vi "WaveGeneratorSelect.vi"(0 "Serial port name":refnum<visa-resource-name>, 2 "start commands":string[](array[string]), 3 "stop commands":string[](array[string])) -> (6 "waveform buffer":T1, 8 "error out":errorcluster)   [LabVIEW 2014]
uses:
  <vilib>/Instr/_visa.llb/VISA Flush IO Buffer Mask.ctl
  <vilib>/Instr/_visa.llb/VISA Configure Serial Port (Instr).vi
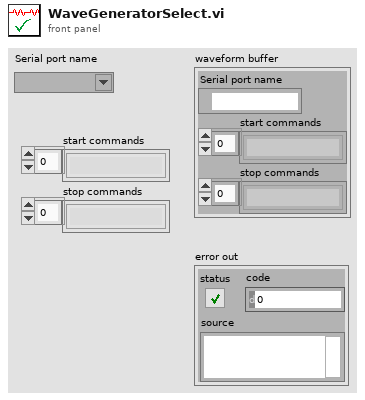
[diagram p1: front panel]
types:
  T1 = cluster{"Serial port name":refnum<visa-resource-name>, "start commands":string[], "stop commands":string[]}
  T2 = typedef "VISA Flush IO Buffer Mask.ctl" = u16
  T3 = cluster{"VISA resource name out":refnum<visa-resource-name>, "start commands":string[], "stop commands":string[]}
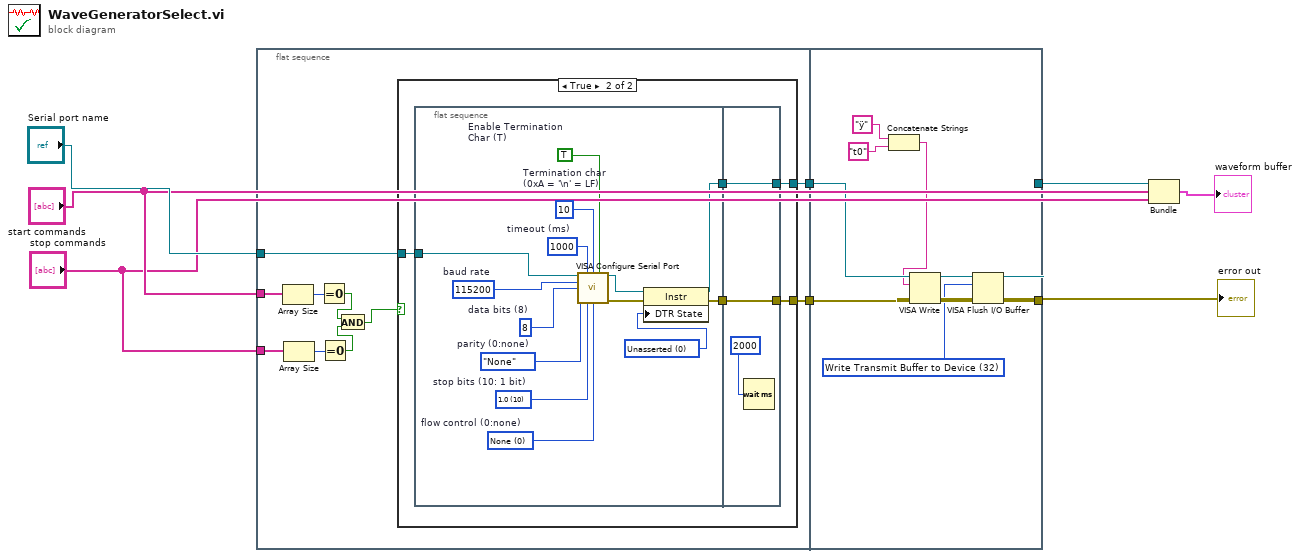
[diagram p0: block diagram]
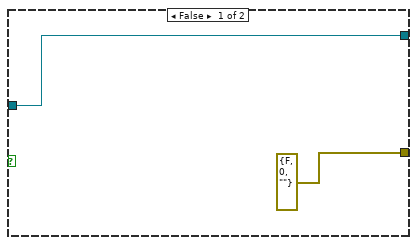
[diagram p2: hidden frame]
diagram:
  n1 = flat-sequence {
    tunnel: "Serial port name" -> [w10]
    tunnel: "start commands" -> [w14]
    tunnel: "stop commands" -> [w13]
    tunnel: [w12] -> w2
    tunnel: [w11] -> w1
    tunnel: [w44] -> w3
    tunnel: [w46] -> w4
    tunnel: w2 -> [w51]
    tunnel: w1 -> [w52]
    frame #0 {
      n2 = Array Size(array=w14) -> (size(s)=w18:i32)
      n3 = Array Size(array=w13) -> (size(s)=w17:i32)
      n4 = Equal To 0?(x=w18) -> (x = 0?=w15:bool)
      n5 = Equal To 0?(x=w17) -> (x = 0?=w16:bool)
      n6 = And(x=w15, y=w16) -> (x .and. y?=w9:bool)
      n7 = case shown="True" w9 {
        tunnel: [w20 w25] -> w12
        tunnel: [errorcluster {"status"=FALSE, "code"=0, "source"=""} ("error constant") w24] -> w11
        tunnel: w10 -> [w20 w23]
        frame False {
        }
        frame True {
          n8 = flat-sequence {
            tunnel: w23 -> [w26]
            tunnel: [w29] -> w22
            tunnel: [w28] -> w21
            tunnel: [w41] -> w24
            tunnel: [w42] -> w25
            tunnel: w22 -> [w42]
            tunnel: w21 -> [w41]
            frame #0 {
              w27 = i16 0 items=["Unknown"=-1, "Unasserted"=0, "Asserted"=1] ("Serial Settings:Modem Line Settings:Line DTR State")
              w32 = TRUE  # Enable Termination Char (T)
              w33 = u8 10  # Termination char (0xA = '\n' = LF)
              w34 = u16 0 items=["None", "XON/XOFF", "RTS/CTS", "XON/XOFF & RTS/CTS", "DTR/DSR", "XON/XOFF & DTR/DSR"]  # flow control (0:none)
              w35 = u16 10 items=["1.0"=10, "1.5"=15, "2.0"=20]  # stop bits (10: 1 bit)
              w36 = u32 1000  # timeout (ms)
              w37 = enum16{"None", "Odd", "Even", "Mark", "Space"}."None"  # parity (0:none)
              w38 = u16 8  # data bits (8)
              w39 = u32 115200  # baud rate
              n9 = call-poly "VISA Configure Serial Port"("VISA resource name"=w26, "timeout (10sec)"=w36, "termination char\n(0xA = '\\n' = LF)"=w33, "Enable Termination\nChar (T)"=w32, "baud rate (9600)"=w39, "data bits (8)"=w38, "parity (0:none)"=w37, "stop bits (10: 1 bit)"=w35, "flow control (0:none)"=w34) -> ("VISA resource name out"=w31:refnum<visa-resource-name>, "error out"=w30:errorcluster)  [unwired: 5 in]
              n10 = property class="Instr"(reference=w31, error in=w30, "DTR State"=w27) -> (reference out=w29:refnum<visa-resource-name>, error out=w28:errorcluster)
            }
            frame #1 {
              n11 = Wait (ms)(milliseconds to wait=u32 2000) -> ()  [unwired: 1 out]
            }
          }
        }
      }
    }
    frame #1 {
      w43 = T2 32 items=["Flush Receive Buffer"=16, "Write Transmit Buffer to Device"=32, "Flush Receive Buffer (No I/O)"=64, "Flush Transmit Buffer"=128] ("Mask")
      n12 = Concatenate Strings("ÿ" ("string"), "t0" ("string")) -> (w50:string)
      n13 = VISA Write(VISA resource name=w51, write buffer=w50, error in (no error)=w52) -> (VISA resource name out=w47:refnum<visa-resource-name>, error out=w45:errorcluster)  [unwired: 1 out]
      n14 = VISA Flush I/O Buffer(VISA resource name=w47, mask (16)=w43, error in (no error)=w45) -> (VISA resource name out=w46:refnum<visa-resource-name>, error out=w44:errorcluster)
    }
  }
  n15 = Bundle("VISA resource name out"=w4, "start commands"="start commands", "stop commands"="stop commands") -> (→"waveform buffer":T3)  [unwired: 1 in]
  "error out" <- w3
